vi "Prueba_movimiento_motor.vi"() -> ()   [LabVIEW 2018]
uses:
  <vilib>/DAQmx/write.llb/DAQmx Write (Digital 1D Bool 1Chan 1Samp).vi
  <vilib>/DAQmx/configure/timing.llb/DAQmx Timing (Implicit).vi
  <vilib>/DAQmx/create/channels.llb/DAQmx Create Channel (DO-Digital Output).vi
  <vilib>/DAQmx/create/channels.llb/DAQmx Create Channel (CO-Pulse Generation-Frequency).vi
  <vilib>/DAQmx/create/channels.llb/DAQmx Create Channel (AI-Voltage-Basic).vi
  <vilib>/DAQmx/write.llb/DAQmx Write (Counter Frequency 1Chan 1Samp).vi
  <vilib>/DAQmx/read.llb/DAQmx Read (Analog DBL 1Chan 1Samp).vi
panel:
  in  "Ancho de pulso":dbl=50.0
  out "Sensor":dbl format="%0.2f V"
  in  "Enable":bool
  in  "frequency":dbl=100.0 caption="Frecuencia PWM" format="%_6g"
  in  "CW":bool
  in  "CCW":bool
  in  "stop":bool
  # "1. Establecer una frecuencia para el tren de pulsos.\n2. Habilitar la salida de PWM.\n3. Dejar presionado el botón CCW o CW para verficar el sentido de giro. Si el sentido no es correcto, cambiar la polaridad del motor.\n4. Verificar la polaridad del potenciómetro. Cambiarla si es necesario."
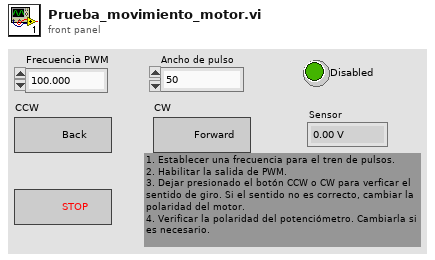
[diagram p1: front panel]
types:
  T1 = enum8{"Enabled", "Disabled", "Disabled and Grayed Out"}
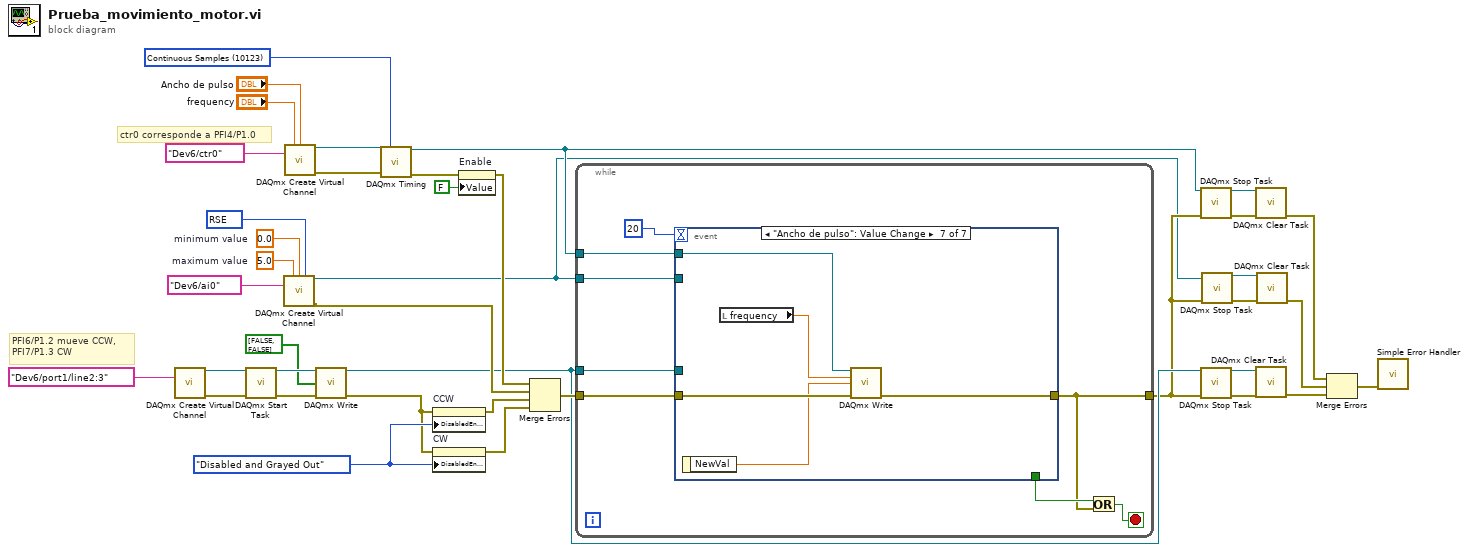
[diagram p0: block diagram]
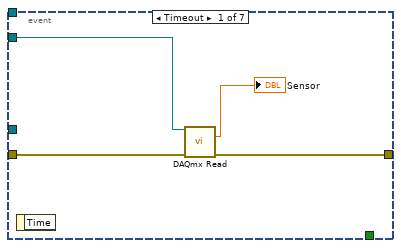
[diagram p2: hidden frame]
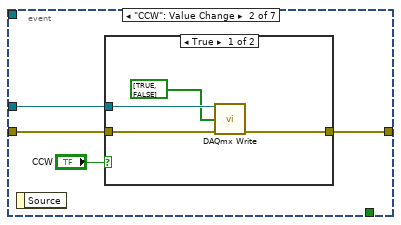
[diagram p3: hidden frame]
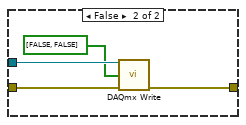
[diagram p4: hidden frame]
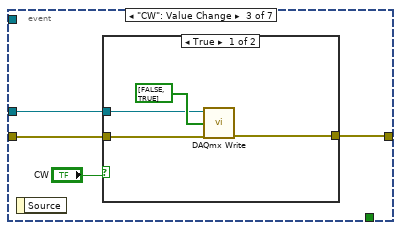
[diagram p5: hidden frame]
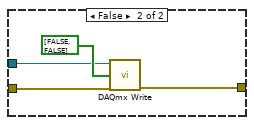
[diagram p6: hidden frame]
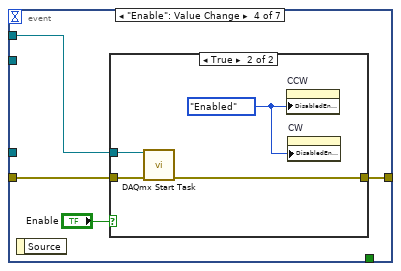
[diagram p7: hidden frame]
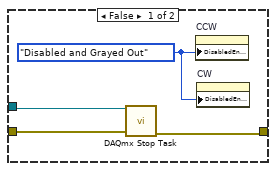
[diagram p8: hidden frame]
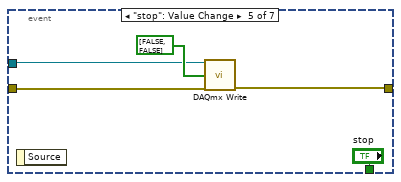
[diagram p9: hidden frame]
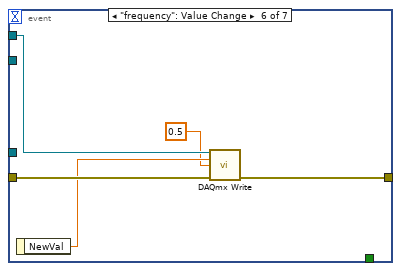
[diagram p10: hidden frame]
diagram:
  w17 = 10083 items=["Default"=-1, "RSE"=10083, "NRSE"=10078, "Differential"=10106, "Pseudodifferential"=12529] ("input terminal configuration")
  w18 = 0.0  # minimum value
  w19 = 5.0  # maximum value
  w22 = T1."Disabled and Grayed Out" ("Disabled")
  w39 = 10123 items=["Finite Samples"=10178, "Continuous Samples"=10123, "Hardware Timed Single Point"=12522] ("sample mode")
  # "PFI6/P1.2 mueve CCW,\nPFI7/P1.3 CW"
  # "ctr0 corresponde a PFI4/P1.0"
  n1 = call-poly <vilib>:"DAQmx Create Virtual Channel.vi"("lines"=tag "Dev6/port1/line2:3") -> ("task out"=w25:refnum<k21>, "error out"=w26:errorcluster)  [unwired: 13 in]
  n2 = call <vilib>:"DAQmx Start Task.vi"("task/channels in"=w25, "error in"=w26) -> ("task out"=w9:refnum<k21>, "error out"=w21:errorcluster)  [unwired: 12 in]
  n3 = call-poly <vilib>:"DAQmx Create Virtual Channel.vi"("maximum value"=w19, "minimum value"=w18, "input terminal configuration"=w17, "physical channels"=tag "Dev6/ai0") -> ("task out"=w1:refnum<k21>, "error out"=w15:errorcluster)  [unwired: 10 in]
  n4 = call-poly <vilib>:"DAQmx Create Virtual Channel.vi"("frequency"="frequency", "duty cycle"="Ancho de pulso", "counter"=tag "Dev6/ctr0") -> ("task out"=w30:refnum<k21>, "error out"=w31:errorcluster)  [unwired: 11 in]
  n5 = call-poly <vilib>:"DAQmx Write.vi"("task/channels in"=w9, "data"=bool[] [FALSE, FALSE], "error in"=w21) -> ("task out"=w8:refnum<k21>, "error out"=w10:errorcluster)  [unwired: 10 in, 1 out]
  n6 = call-poly <vilib>:"DAQmx Timing.vi"("task/channels in"=w30, "sample mode"=w39, "error in"=w31) -> ("task out"=w11:refnum<k21>, "error out"=w24:errorcluster)  [unwired: 11 in]
  n7 = property on="CCW" class="Bool (strict)"(error in=w10, "DisabledEnum"=w22) -> (error out=w14:errorcluster)  [unwired: 1 in, 1 out]
  n8 = property on="CW" class="Bool (strict)"(error in=w10, "DisabledEnum"=w22) -> (error out=w13:errorcluster)  [unwired: 1 in, 1 out]
  n9 = property on="Enable" class="Bool (strict)"(error in=w24, "Value"=FALSE ("Enable")) -> (error out=w16:errorcluster)  [unwired: 1 in, 1 out]
  n10 = Merge Errors(w16, w15, w14, w13) -> (w12:errorcluster)
  n11 = while {
    tunnel: w11 -> [w45]
    tunnel: w8 -> [w44]
    tunnel: w12 -> [w47]
    tunnel: [w42] -> w5
    tunnel: w1 -> [w41]
    stop <- w43 stop-if-true
    n12 = event shown="[6] \"Ancho de pulso\": Value Change" {
      selector: _ -> [_ _ _ _ _ _ _]
      dyn-events: _ -> [_ _ _ _ _ _ _]
      timeout: 20 -> [_ _ _ _ _ _ _]
      tunnel: w47 -> [w51 w55 w67 w79 w90 w97 w102]
      tunnel: [w50 w54 w66 w78 w88 w96 w101] -> w42
      tunnel: [_ _ _ _ "stop" _ _] -> w46
      tunnel: w45 -> [_ _ _ w77 _ w95 w100]
      tunnel: w44 -> [_ w53 w65 _ w89 _ _]
      tunnel: w41 -> [w49 _ _ _ _ _ _]
      event Timeout {
        n13 = event-data() -> ()  [unwired: 1 in, 1 out]
        n14 = call-poly <vilib>:"DAQmx Read.vi"("task/channels in"=w49, "error in"=w51) -> ("data"=→"Sensor":dbl, "error out"=w50:errorcluster)  [unwired: 11 in, 1 out]
      }
      event "CCW": Value Change {
        n15 = event-data() -> ()  [unwired: 1 in, 1 out]
        n16 = case shown="True" "CCW" {
          tunnel: w55 -> [w59 w63]
          tunnel: [w58 w62] -> w54
          tunnel: w53 -> [w57 w61]
          frame True {
            n17 = call-poly <vilib>:"DAQmx Write.vi"("task/channels in"=w57, "data"=bool[] [TRUE, FALSE], "error in"=w59) -> ("error out"=w58:errorcluster)  [unwired: 10 in, 2 out]
          }
          frame False {
            n18 = call-poly <vilib>:"DAQmx Write.vi"("task/channels in"=w61, "data"=bool[] [FALSE, FALSE], "error in"=w63) -> ("error out"=w62:errorcluster)  [unwired: 10 in, 2 out]
          }
        }
      }
      event "CW": Value Change {
        n19 = event-data() -> ()  [unwired: 1 in, 1 out]
        n20 = case shown="True" "CW" {
          tunnel: w67 -> [w70 w74]
          tunnel: [w69 w73] -> w66
          tunnel: w65 -> [w68 w72]
          frame True {
            n21 = call-poly <vilib>:"DAQmx Write.vi"("task/channels in"=w68, "data"=bool[] [FALSE, TRUE], "error in"=w70) -> ("error out"=w69:errorcluster)  [unwired: 10 in, 2 out]
          }
          frame False {
            n22 = call-poly <vilib>:"DAQmx Write.vi"("task/channels in"=w72, "data"=bool[] [FALSE, FALSE], "error in"=w74) -> ("error out"=w73:errorcluster)  [unwired: 10 in, 2 out]
          }
        }
      }
      event "Enable": Value Change {
        n23 = event-data() -> ()  [unwired: 1 in, 1 out]
        n24 = case shown="True" "Enable" {
          tunnel: w79 -> [w83 w87]
          tunnel: [w81 w85] -> w78
          tunnel: w77 -> [w82 w86]
          frame False {
            w80 = T1."Disabled and Grayed Out" ("Disabled")
            n25 = call <vilib>:"DAQmx Stop Task.vi"("task/channels in"=w82, "error in"=w83) -> ("error out"=w81:errorcluster)  [unwired: 12 in, 1 out]
            n26 = property on="CCW" class="Bool (strict)"("DisabledEnum"=w80) -> ()  [unwired: 2 in, 2 out]
            n27 = property on="CW" class="Bool (strict)"("DisabledEnum"=w80) -> ()  [unwired: 2 in, 2 out]
          }
          frame True {
            w84 = T1."Enabled" ("Disabled")
            n28 = call <vilib>:"DAQmx Start Task.vi"("task/channels in"=w86, "error in"=w87) -> ("error out"=w85:errorcluster)  [unwired: 12 in, 1 out]
            n29 = property on="CCW" class="Bool (strict)"("DisabledEnum"=w84) -> ()  [unwired: 2 in, 2 out]
            n30 = property on="CW" class="Bool (strict)"("DisabledEnum"=w84) -> ()  [unwired: 2 in, 2 out]
          }
        }
      }
      event "stop": Value Change {
        n31 = event-data() -> ()  [unwired: 1 in, 1 out]
        n32 = call-poly <vilib>:"DAQmx Write.vi"("task/channels in"=w89, "data"=bool[] [FALSE, FALSE], "error in"=w90) -> ("error out"=w88:errorcluster)  [unwired: 10 in, 2 out]
      }
      event "frequency": Value Change {
        n33 = event-data() -> ("NewVal"=w94:dbl)  [unwired: 1 in]
        n34 = call-poly <vilib>:"DAQmx Write.vi"("task/channels in"=w95, "frequency"=w94, "duty cycle"=0.5, "error in"=w97) -> ("error out"=w96:errorcluster)  [unwired: 9 in, 2 out]
      }
      event "Ancho de pulso": Value Change {
        n35 = event-data() -> ("NewVal"=w98:dbl)  [unwired: 1 in]
        n36 = local read "frequency"() -> (w99:dbl)
        n37 = call-poly <vilib>:"DAQmx Write.vi"("task/channels in"=w100, "frequency"=w99, "duty cycle"=w98, "error in"=w102) -> ("error out"=w101:errorcluster)  [unwired: 9 in, 2 out]
      }
    }
    n38 = Or(x=w46, y=w42) -> (x .or. y?=w43:bool)
  }
  n39 = call <vilib>:"DAQmx Stop Task.vi"("task/channels in"=w11, "error in"=w5) -> ("task out"=w38:refnum<k21>, "error out"=w37:errorcluster)  [unwired: 12 in]
  n40 = call <vilib>:"DAQmx Stop Task.vi"("task/channels in"=w8, "error in"=w5) -> ("task out"=w36:refnum<k21>, "error out"=w35:errorcluster)  [unwired: 12 in]
  n41 = call <vilib>:"DAQmx Stop Task.vi"("task/channels in"=w1, "error in"=w5) -> ("task out"=w2:refnum<k21>, "error out"=w4:errorcluster)  [unwired: 12 in]
  n42 = call <vilib>:"DAQmx Clear Task.vi"("task in"=w38, "error in"=w37) -> ("error out"=w33:errorcluster)  [unwired: 13 in]
  n43 = call <vilib>:"DAQmx Clear Task.vi"("task in"=w36, "error in"=w35) -> ("error out"=w34:errorcluster)  [unwired: 13 in]
  n44 = call <vilib>:"DAQmx Clear Task.vi"("task in"=w2, "error in"=w4) -> ("error out"=w3:errorcluster)  [unwired: 13 in]
  n45 = Merge Errors(w33, w3, w34) -> (w32:errorcluster)
  n46 = call <vilib>:"Simple Error Handler.vi"("error in (no error)"=w32) -> ()  [unwired: 4 in, 5 out]
